vi "Load Instruments names.vi"(8 "error in (no error)":errorcluster, 11 "Test Framework in":refnum<class "Test Framework.lvclass">) -> (0 "error out":errorcluster, 3 "Test Framework out":refnum<class "Test Framework.lvclass">)   [LabVIEW 2020, in "Test Framework.lvclass"]
uses:
  Test Framework.lvclass
  Instruments/Instrument.lvclass
  Test Framework.lvclass/Test Framework.ctl
  <vilib>/Utility/xml.llb/Read From XML File(string).vi
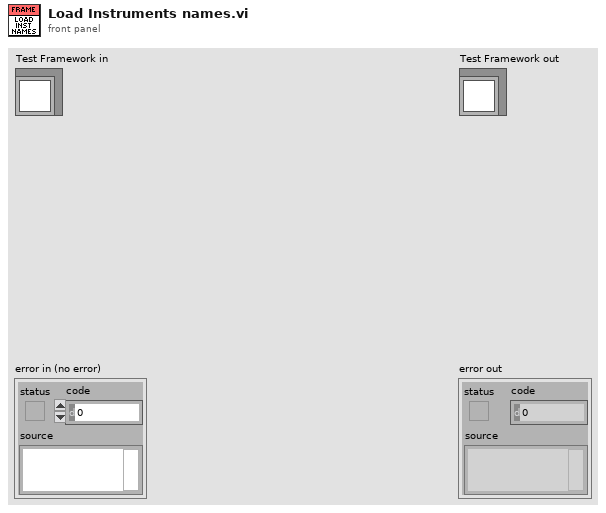
[diagram p1: front panel]
types:
  T1 = cluster{"Instrument Name":string, "Instrument.lvclass":refnum<class "Instrument.lvclass">, "Reference":bool}
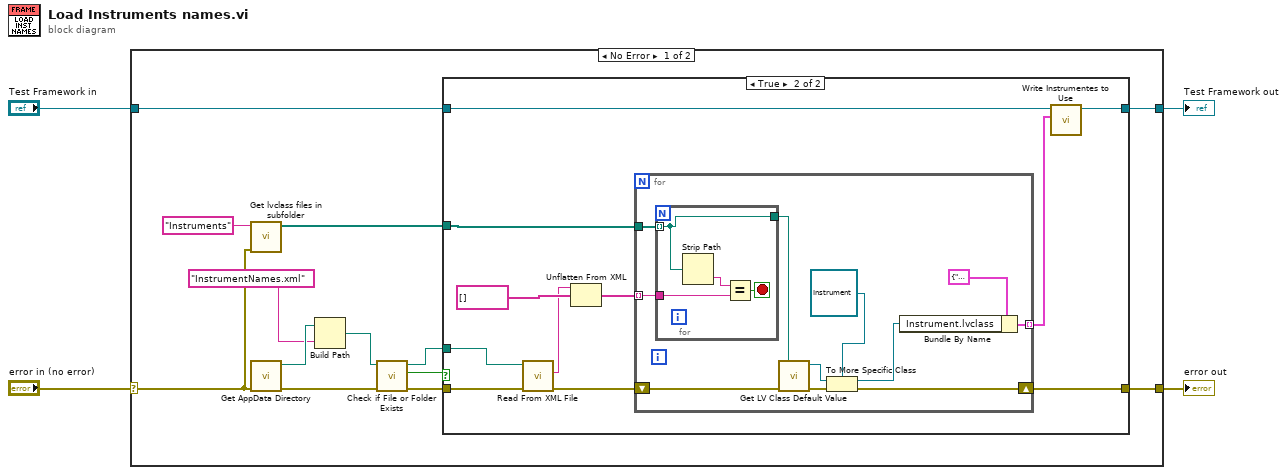
[diagram p0: block diagram]
diagram:
  n1 = case shown="No Error" "error in (no error)" {
    selector: "error in (no error)" -> [w17 w47]
    tunnel: [w5 w47] -> w3
    tunnel: [w6 w46] -> w1
    tunnel: "Test Framework in" -> [w7 w46]
    frame No Error {
      n2 = call "Get lvclass files in subfolder.vi"("Error In"=w17, "Sub Folder"="Instruments") -> ("Found lvclass files"=w8:path[])  [unwired: 8 in, 1 out]
      n3 = call "Get AppData Directory.vi"("Error In"=w17) -> ("Error Out"=w13:errorcluster, "Folder path"=w15:path)  [unwired: 8 in, 1 out]
      n4 = Build Path(base path=w15, name or relative path="InstrumentNames.xml") -> (appended path=w12:path)
      n5 = call <vilib>:"Check if File or Folder Exists.vi"("error in (no error)"=w13, "path"=w12) -> ("error out"=w10:errorcluster, "file or folder exists?"=w11:bool, "dup path"=w9:path)  [unwired: 7 in]
      n6 = case shown="True" w11 {
        tunnel: w10 -> [w18 w30]
        tunnel: w9 -> [_ w29]
        tunnel: w8 -> [_ w26]
        tunnel: w7 -> [w19 w23]
        tunnel: [w19 w22] -> w6
        tunnel: [w18 w20] -> w5
        frame False {
        }
        frame True {
          n7 = call-poly <vilib>:"Read From XML File.vi"("error in (no error)"=w30, "XML File Path"=w29) -> ("error out"=w24:errorcluster, "XML Elements"=w27:string)  [unwired: 7 in, 1 out]
          n8 = Unflatten From XML(xml string=w27, type=string[] []) -> (value=w25:string[])  [unwired: 1 in, 1 out]
          n9 = for {
            tunnel: w26 -> [w40]
            tunnel: w25 -> [w41] mode=indexing
            shift-right: [w35] -> w20
            shift-left: w24 -> [w38]
            tunnel: [w32] -> w21 mode=indexing
            n10 = for {
              tunnel: w41 -> [w44]
              tunnel: w40 -> [w42] mode=indexing
              tunnel: [w42] -> w39
              stop <- w43 stop-if-true
              n11 = Strip Path(path=w42) -> (name=w45:string)  [unwired: 1 out]
              n12 = Equal?(x=w45, y=w44) -> (x = y?=w43:bool)
            }
            n13 = call <vilib>:"Get LV Class Default Value.vi"("error in (no error)"=w38, "class path"=w39) -> ("error out"=w36:errorcluster, "object"=w37:refnum<class>)  [unwired: 8 in]
            n14 = To More Specific Class(target class=refnum<class "Instrument.lvclass"> refnum ("Instrument.lvclass"), reference=w37, error in=w36) -> (specific class reference=w33:refnum<class "Instrument.lvclass">, error out=w35:errorcluster)
            n15 = Bundle By Name(cluster=T1 {"Instrument Name"="", "Instrument.lvclass"=refnum, "Reference"=FALSE} ("Instrument to Use"), "Instrument.lvclass"=w33) -> (w32:T1)
          }
          n16 = call "Write Instrumentes to Use.vi"("Instruments to Use"=w21, "Test Framework in"=w23) -> ("Test Framework out"=w22:refnum<class "Test Framework.lvclass">)  [unwired: 9 in]
        }
      }
    }
    frame Error {
    }
  }
  "error out" <- w3
  "Test Framework out" <- w1
